vi "DE - Enable-disable data acquisition.vi"(1 "Enable/disable the data acquisition request\nTo enable enter a 1\nTo disable enter a 0":dbl format="%.2f", 2 "error in":errorcluster, 3 "Address / Port":i16=1 min=1 max=31 step=1) -> (0 "error out":errorcluster)   [LabVIEW 2014]
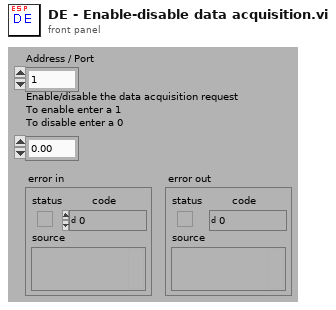
[diagram p1: front panel]
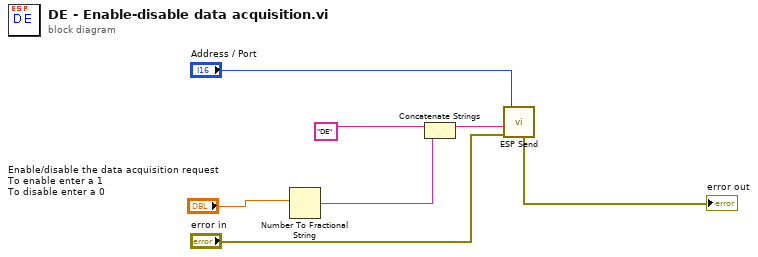
[diagram p0: block diagram]
diagram:
  n1 = Number To Fractional String(number="Enable/disable the data acquisition request\nTo enable enter a 1\nTo disable enter a 0") -> (F-format string=w1:string)  [unwired: 3 in]
  n2 = Concatenate Strings("DE" ("Substring"), w1) -> (w6:string)
  n3 = call "ESP Send.vi"("Address / Port"="Address / Port", "Command String"=w6, "error in"="error in") -> ("error out"=→"error out":errorcluster)  [unwired: 5 in]
